vi "HEWH Find Qr and Tmax1.vi"(7 "Water Heater Type":T6, 8 "error in (no error)":errorcluster, 11 "UEF Calculated Values":T1 {"Data Indexes"."15 sec after Draw Index" format="%#.2f"; "Data Indexes"."15 sec after Draw Timestamp" format="%#.2f"; "Data Indexes"."Test Start Timestamp" format="%.2f"; "Data Indexes"."Test End Timestamp" format="%.2f"; "Data Indexes"."T0 Timestamp" format="%.2f"; "Data Indexes"."Tsf Timestamp" format="%.2f"; "Data Indexes"."Tsu0 Timestamp" format="%.2f"; "Data Indexes"."Tmax1 Timestamp" format="%.2f"; "Data Indexes"."Draw Index Timestamp" format="%#.2f"; "Data Indexes"."Non-Draw Timestamp" format="%#.2f"; "Data Indexes"."Heating Timestamp" format="%#.2f"; "Data Indexes"."Start Energy (BTU-Gas)" format="%.6f"; "Data Indexes"."Start Watt Hours" format="%.6f"; "Static Data"."V - Volume of Wh (True)" format="%.5f"; "Static Data"."T-Ambinet Nominal (°F)" format="%.5f"; "Static Data"."T-Inlet Setpoint (°F)" format="%.5f"; "Static Data"."T-Wh Setpoint (°F)" format="%.5f"; "Sampled Data"."Qe (Wh)" format="%.5f"; "Sampled Data"."Tau stby2 (hr)" format="%.5f"; "Sampled Data"."Tastby2 (°F)" format="%.5f"; "Sampled Data"."Qf (BTU)" format="%.5f"; "Sampled Data"."Qe (BTU)" format="%.5f"; "Sampled Data"."Tmax1 (°F)" format="%.5f"; "Sampled Data"."T0 (°F)" format="%.5f"; "Sampled Data"."Qr (BTU)" format="%.5f"; "Sampled Data"."T 24(°F)" format="%.5f"; "Sampled Data"."T astby(°F)" format="%.5f"; "Sampled Data"."T tstby(°F)" format="%.5f"; "Sampled Data"."T su0(°F)" format="%.5f"; "Sampled Data"."T suf(°F)" format="%.5f"; "Sampled Data"."Tau stby_1 (hr)" format="%.5f"; "Sampled Data"."Qsuf (BTU)" format="%.5f"; "Sampled Data"."Qsu0 (BTU)" format="%.5f"; "Calculated Values"."Draw Bonus Volume (gal)" format="%.6f"; "Calculated Values"."Adjustment Factor" format="%.6f"; "Calculated Values"."T*avg_del(n-1)" format="%.6f"; "Calculated Values"."T*min(n-1)" format="%.6f"; "Calculated Values"."T*avg_del(n)" format="%.6f"; "Calculated Values"."Vn" format="%.6f"; "Calculated Values"."Qdm (BTU)" format="%.6f"; "Calculated Values"."QHWD (BTU)" format="%.6f"; "Calculated Values"."QHW (BTU)" format="%.6f"; "Calculated Values"."UEF" format="%.6f"; "Calculated Values"."QHW67 (BTU)" format="%.6f"; "Calculated Values"."Qda (BTU)" format="%.6f"; "Calculated Values"."Qd (BTU)" format="%.6f"; "Calculated Values"."Q (BTU)" format="%.6f"; "Calculated Values"."UA (BTU/(hr*F))" format="%.6f"; "Calculated Values"."Qhr (BTU/hr)" format="%.6f"; "Calculated Values"."Qstby (BTU)" format="%.6f"; "Calculated Values"."nu_r" format="%.6f"; "Calculated Values"."CpUEF (BTU/(lb*F))" format="%.6f"; "Calculated Values"."rho_nu (lb/gal)" format="%.6f"; "Calculated Values"."V1- Vol (Gal)" format="%.6f"; "Calculated Values"."M cluster mass removed (lb)" format="%.6f"; "Calculated Values"."Cp theoretical (BTU/(lbm °F))" format="%.6f"; "Calculated Values"."Tin1 - Mean Inlet 1st Cluster (°F)" format="%.6f"; "Calculated Values"."Tdel1-Mean Outlet 1st Cluster(°F)" format="%.6f"; "Calculated Values"."Cp 24 (BTU/(lb*F))" format="%.6f"; "Calculated Values"."Cp standby (BTU/(lb*F))" format="%.6f"; "Calculated Values"."Cp2 (BTU/(lb*F))" format="%.6f"; "Calculated Values"."Cp1 (BTU/(lb*F))" format="%.6f"; "Calculated Values"."rho 24 (lb/gal)" format="%.6f"; "Calculated Values"."rho standby (lb/gal)" format="%.6f"; "Calculated Values"."rho 2 (lb/gal)" format="%.6f"; "Calculated Values"."Density of cold water All (lbm/gal)" format="%#.3g"; "Calculated Values"."CpHW (BTU/(lbm °F))" format="%#.3g"; "Calculated Values"."Density of hot water All (lbm/gal)" format="%#.3g"; "Calculated Values"."Mass of water All (lbm)" format="%#.3f"}) -> (0 "error out":errorcluster, 3 "UEF Calculated Values Output":T1={"Calculated Values"={"Draw Cluster - Actual (Gal)"=[], "Mass of water All (lbm)"=[], "Density of hot water All (lbm/gal)"=[], "CpHW (BTU/(lbm °F))"=[], "rho 2 (lb/gal)"=0.0, "rho standby (lb/gal)"=0.0, "rho 24 (lb/gal)"=0.0, "Cp1 (BTU/(lb*F))"=0.0, "Cp2 (BTU/(lb*F))"=0.0, "Cp standby (BTU/(lb*F))"=0.0, "Cp 24 (BTU/(lb*F))"=0.0, "nu_r"=0.0, "Qstby (BTU)"=0.0, "Qhr (BTU/hr)"=0.0, "UA (BTU/(hr*F))"=0.0, "Q (BTU)"=0.0, "Qd (BTU)"=0.0, "Qda (BTU)"=0.0, "QHW67 (BTU)"=0.0, "UEF"=0.0, "Tdel1-Mean Outlet 1st Cluster(°F)"=0.0, "Tin1 - Mean Inlet 1st Cluster (°F)"=0.0, "Cp theoretical (BTU/(lbm °F))"=0.0, "M cluster mass removed (lb)"=0.0, "V1- Vol (Gal)"=0.0, "Test Data -Start to End (Full Index)"=[], "rho_nu (lb/gal)"=0.0, "Density of cold water All (lbm/gal)"=[], "CpUEF (BTU/(lb*F))"=0.0, "QHW (BTU)"=0.0, "QHWD (BTU)"=0.0, "Qdm (BTU)"=0.0, "FHD-After 1 Hour (String)"=[], "Vn"=0.0, "T*avg_del(n)"=0.0, "Max Location"=0, "T*min(n-1)"=0.0, "T*avg_del(n-1)"=0.0, "Temp Greater than T*min(n-1)"=FALSE, "Adjustment Factor"=0.0, "Draw Bonus Volume (gal)"=0.0, "Flow Type - End Condition"=enum."ForcedDrawAfterHour"}, "Sampled Data"={"Cold Water Draw Amounts-(Gal)"=[14.98, 1.97, 9.0, 8.97, 4.98, 0.98, 0.96, 0.96, 0.96, 1.96, 1.99, 6.98], "T del_all - Outlet Temps (°F)"=[121.5, 121.3, 124.5, 120.0, 121.2, 120.1, 119.0, 120.3, 116.6, 118.8, 118.3, 118.3], "T in_all - Inlet Temps (°F)"=[58.5, 58.2, 58.4, 58.6, 58.6, 58.1, 58.1, 58.3, 56.3, 58.5, 58.5, 58.5], "Qsu0 (BTU)"=9772.3, "Qsuf (BTU)"=9773.0, "Tau stby_1 (hr)"=6.7, "T suf(°F)"=107.7, "T su0(°F)"=109.3, "T tstby(°F)"=108.5, "T astby(°F)"=68.2, "T 24(°F)"=117.9, "Qr (BTU)"=7628.5, "T0 (°F)"=121.1, "Tmax1 (°F)"=122.4, "Qe (BTU)"=29606.3, "Qf (BTU)"=0.0, "Tastby2 (°F)"=68.3, "RTD Out Full Data\nSet (Each Draw)"=[], "RTD IN Full Data\nSet (Each Draw)"=[], "Tau stby2 (hr)"=23.406, "Hot Water Draw Amounts-(Gal)"=[], "Cold Flow Rate (GPM)"=[], "Hot Flow Rate (GPM)"=[], "Softw Elapsed Time\n Full Data Set (Each Draw)"=[], "Cold Gal Total Full\nData Set (Each Draw)"=[], "Total Hot Draw Amount (Gal) "=0.0, "Total Cold Draw Amount (Gal)"=0.0, "Qe (Wh)"=0.0, "Hot Gal Total Full\nData Set (Each Draw)"=[]}, "Static Data"={"T-Wh Setpoint (°F)"=125.0, "T-Inlet Setpoint (°F)"=58.0, "T-Ambinet Nominal (°F)"=67.5, "V - Volume of Wh (True)"=46.0}, "Data Indexes"={"Test Start-Full Index (Found)"=0, "Header Length"=0, "Draw Index (Found)"=[], "Nr"=0, "Start Watt Hours"=0.0, "Tsu0 Index (Found)"=0, "Tsf Index (Found)"=0, "Start Energy (BTU-Gas)"=0.0, "Draws in Cluster"=0, "T0 Index-Full Index (Found)"=0, "Non-Draw Index (Found)"=[], "Tmax1 Index (Found)"=0, "Test End-Full Index (Found)"=0, "Heating Index (Found)"=[], "Heating Timestamp"=[], "Non-Draw Timestamp"=[], "Draw Index Timestamp"=[], "Tmax1 Timestamp"=0.0, "Tsu0 Timestamp"=0.0, "Tsf Timestamp"=0.0, "T0 Timestamp"=0.0, "Test End Timestamp"=0.0, "Test Start Timestamp"=0.0, "15 sec after Draw Timestamp"=[], "15 sec after Draw Index"=[], "Tmax1 Occurred During a Draw"=FALSE, "FHD Total Time (Sec)"=0.0, "Draw Pattern"=enum."Very Small Usage", "Standby Valid"=FALSE}, "Raw Data"={"Elapsed Time Index (DBL)"=0, "Software Elapsed Time Index (DBL)"=0, "TC Tree Avg Index (DBL)"=0, "Watt Hours -Wh Index (DBL)"=0, "Energy BTU Index (DBL)"=0, "Totalized Flow Index (DBL)"=0, "Flow Rate Index (DBL)"=0, "Program Status Index (Str)"=0, "RTDin Index (DBL)"=0, "RTDout Index (DBL)"=0, "RTDamb Index (DBL)"=0, "Test Data-Start to End DBL"=[], "Data Type"=enum."GEA Inlet Side Meter", "Heat Source Index (DBL)"=0, "Hot Water Rate GPM (DBL)"=0, "Hot Water Total - GAL (DBL)"=0, "FHD-After 1 hour"=[], "Humidity -% RH (DBL)"=0, "Voltage - V (DBL)"=0, "Draw Count (DBL)"=0, "Elapsed Time Index (Str)"=0, "Software Elapsed Time Index (Str)"=0, "Frequency-Hz (Str)"=0, "RTDin Index (Str)"=0, "RTDout Index (Str)"=0, "RTDamb Index (Str)"=0, "UE (Str)"=0, "LE (Str)"=0, "Compressor (Str)"=0, "Flow Rate Index (Str)"=0, "Hot Water Total - GAL (Str)"=0}, "Tolerance Check (T)=Pass"={"Flow Rate"=FALSE, "Totalized Flow"=FALSE, "Ambient Temp (Full Range)"=FALSE, "Ambient Humidity (Full Range)"=FALSE, "Inlet Temp"=FALSE, "Outlet Temp"=FALSE, "Valid Test"=FALSE, "Individual Totalized Flow"=FALSE, "Data Sheet Check"="", "Inlet Temperature"=[], "Tinlet Max"=[], "Tinlet Min"=[], "Flow Rate Max (Tol)"=[], "Flow Rate Min (Tol)"=[], "Amb Temp Max"=0.0, "Amb Temp Min"=0.0, "Toutlet Max - Draw 1"=0.0, "Humidity Upper Tolerance (%)"=0.0, "Total Volume Tolerance (Gal)"=0.0, "Humidity Lower Tolerance (%)"=0.0, "Flow Rate Max\nPer Draw"=[], "Flow Rate Min\nPer Draw"=[], "Ambient Humidity (Runtime)"=FALSE, "Humidity Avg (Runtime)"=0.0, "Ambient Temp (On-Time AVG)"=FALSE, "Ambient Temp (Off-Time AVG)"=FALSE, "Amb Temp OFF Avg"=0.0, "Amb Temp ON Avg"=0.0, "Voltage (Heating)"=FALSE, "Voltage (Min)"=0.0, "Voltage (Max)"=0.0, "Toutlet Max"=[], "Toutlet Min"=[], "Test_Avg_Outlet_Temp"=0.0}, "Test Information"={"TR Number"="", "Lab ID"="", "Notes/Config"="", "Model Number"="", "Serial Number"="", "Lab Technician"="", "Engineer"="", "Type of Fuel"="", "Samp Received Date"="", "Samp Test Date"="", "Report Date"="", "Rate Input (kW or BTU/hr)"="", "Measured Input (kW or BTU/hr)"="", "Filename"="", "Calibration Information"=[], "Calculator Version"="", "Minimum UEF Per CFR"=0.0, "UEF Report Information"=[], "FHR Report Information"=[], "FHR Front Panel Display"=[], "UEF Front Panel Display"=[], "Draw Outlet Temp Viewer"=[]}} {"Data Indexes"."15 sec after Draw Index" format="%#.2f"; "Data Indexes"."15 sec after Draw Timestamp" format="%#.2f"; "Data Indexes"."Test Start Timestamp" format="%.2f"; "Data Indexes"."Test End Timestamp" format="%.2f"; "Data Indexes"."T0 Timestamp" format="%.2f"; "Data Indexes"."Tsf Timestamp" format="%.2f"; "Data Indexes"."Tsu0 Timestamp" format="%.2f"; "Data Indexes"."Tmax1 Timestamp" format="%.2f"; "Data Indexes"."Draw Index Timestamp" format="%#.2f"; "Data Indexes"."Non-Draw Timestamp" format="%#.2f"; "Data Indexes"."Heating Timestamp" format="%#.2f"; "Data Indexes"."Start Energy (BTU-Gas)" format="%.6f"; "Data Indexes"."Start Watt Hours" format="%.6f"; "Static Data"."V - Volume of Wh (True)" format="%.5f"; "Static Data"."T-Ambinet Nominal (°F)" format="%.5f"; "Static Data"."T-Inlet Setpoint (°F)" format="%.5f"; "Static Data"."T-Wh Setpoint (°F)" format="%.5f"; "Sampled Data"."Qe (Wh)" format="%.5f"; "Sampled Data"."Tau stby2 (hr)" format="%.5f"; "Sampled Data"."Tastby2 (°F)" format="%.5f"; "Sampled Data"."Qf (BTU)" format="%.5f"; "Sampled Data"."Qe (BTU)" format="%.5f"; "Sampled Data"."Tmax1 (°F)" format="%.5f"; "Sampled Data"."T0 (°F)" format="%.5f"; "Sampled Data"."Qr (BTU)" format="%.5f"; "Sampled Data"."T 24(°F)" format="%.5f"; "Sampled Data"."T astby(°F)" format="%.5f"; "Sampled Data"."T tstby(°F)" format="%.5f"; "Sampled Data"."T su0(°F)" format="%.5f"; "Sampled Data"."T suf(°F)" format="%.5f"; "Sampled Data"."Tau stby_1 (hr)" format="%.5f"; "Sampled Data"."Qsuf (BTU)" format="%.5f"; "Sampled Data"."Qsu0 (BTU)" format="%.5f"; "Calculated Values"."Draw Bonus Volume (gal)" format="%.6f"; "Calculated Values"."Adjustment Factor" format="%.6f"; "Calculated Values"."T*avg_del(n-1)" format="%.6f"; "Calculated Values"."T*min(n-1)" format="%.6f"; "Calculated Values"."T*avg_del(n)" format="%.6f"; "Calculated Values"."Vn" format="%.6f"; "Calculated Values"."Qdm (BTU)" format="%.6f"; "Calculated Values"."QHWD (BTU)" format="%.6f"; "Calculated Values"."QHW (BTU)" format="%.6f"; "Calculated Values"."UEF" format="%.6f"; "Calculated Values"."QHW67 (BTU)" format="%.6f"; "Calculated Values"."Qda (BTU)" format="%.6f"; "Calculated Values"."Qd (BTU)" format="%.6f"; "Calculated Values"."Q (BTU)" format="%.6f"; "Calculated Values"."UA (BTU/(hr*F))" format="%.6f"; "Calculated Values"."Qhr (BTU/hr)" format="%.6f"; "Calculated Values"."Qstby (BTU)" format="%.6f"; "Calculated Values"."nu_r" format="%.6f"; "Calculated Values"."CpUEF (BTU/(lb*F))" format="%.6f"; "Calculated Values"."rho_nu (lb/gal)" format="%.6f"; "Calculated Values"."V1- Vol (Gal)" format="%.6f"; "Calculated Values"."M cluster mass removed (lb)" format="%.6f"; "Calculated Values"."Cp theoretical (BTU/(lbm °F))" format="%.6f"; "Calculated Values"."Tin1 - Mean Inlet 1st Cluster (°F)" format="%.6f"; "Calculated Values"."Tdel1-Mean Outlet 1st Cluster(°F)" format="%.6f"; "Calculated Values"."Cp 24 (BTU/(lb*F))" format="%.6f"; "Calculated Values"."Cp standby (BTU/(lb*F))" format="%.6f"; "Calculated Values"."Cp2 (BTU/(lb*F))" format="%.6f"; "Calculated Values"."Cp1 (BTU/(lb*F))" format="%.6f"; "Calculated Values"."rho 24 (lb/gal)" format="%.6f"; "Calculated Values"."rho standby (lb/gal)" format="%.6f"; "Calculated Values"."rho 2 (lb/gal)" format="%.6f"; "Calculated Values"."Density of cold water All (lbm/gal)" format="%#.3g"; "Calculated Values"."CpHW (BTU/(lbm °F))" format="%#.3g"; "Calculated Values"."Density of hot water All (lbm/gal)" format="%#.3g"; "Calculated Values"."Mass of water All (lbm)" format="%#.3f"})   [LabVIEW 2023]
uses:
  Type Definitions/UEF Constants.ctl
  Type Definitions/HEWH Draw Stats.ctl
  Type Definitions/HEWH FHR Draw Type.ctl
  Type Definitions/FHR Bins.ctl
  Type Definitions/HEWH Meter Type.ctl
  Type Definitions/HEWH Water Heater Type.ctl
panel:
  # "FHR"
  # "FHR"
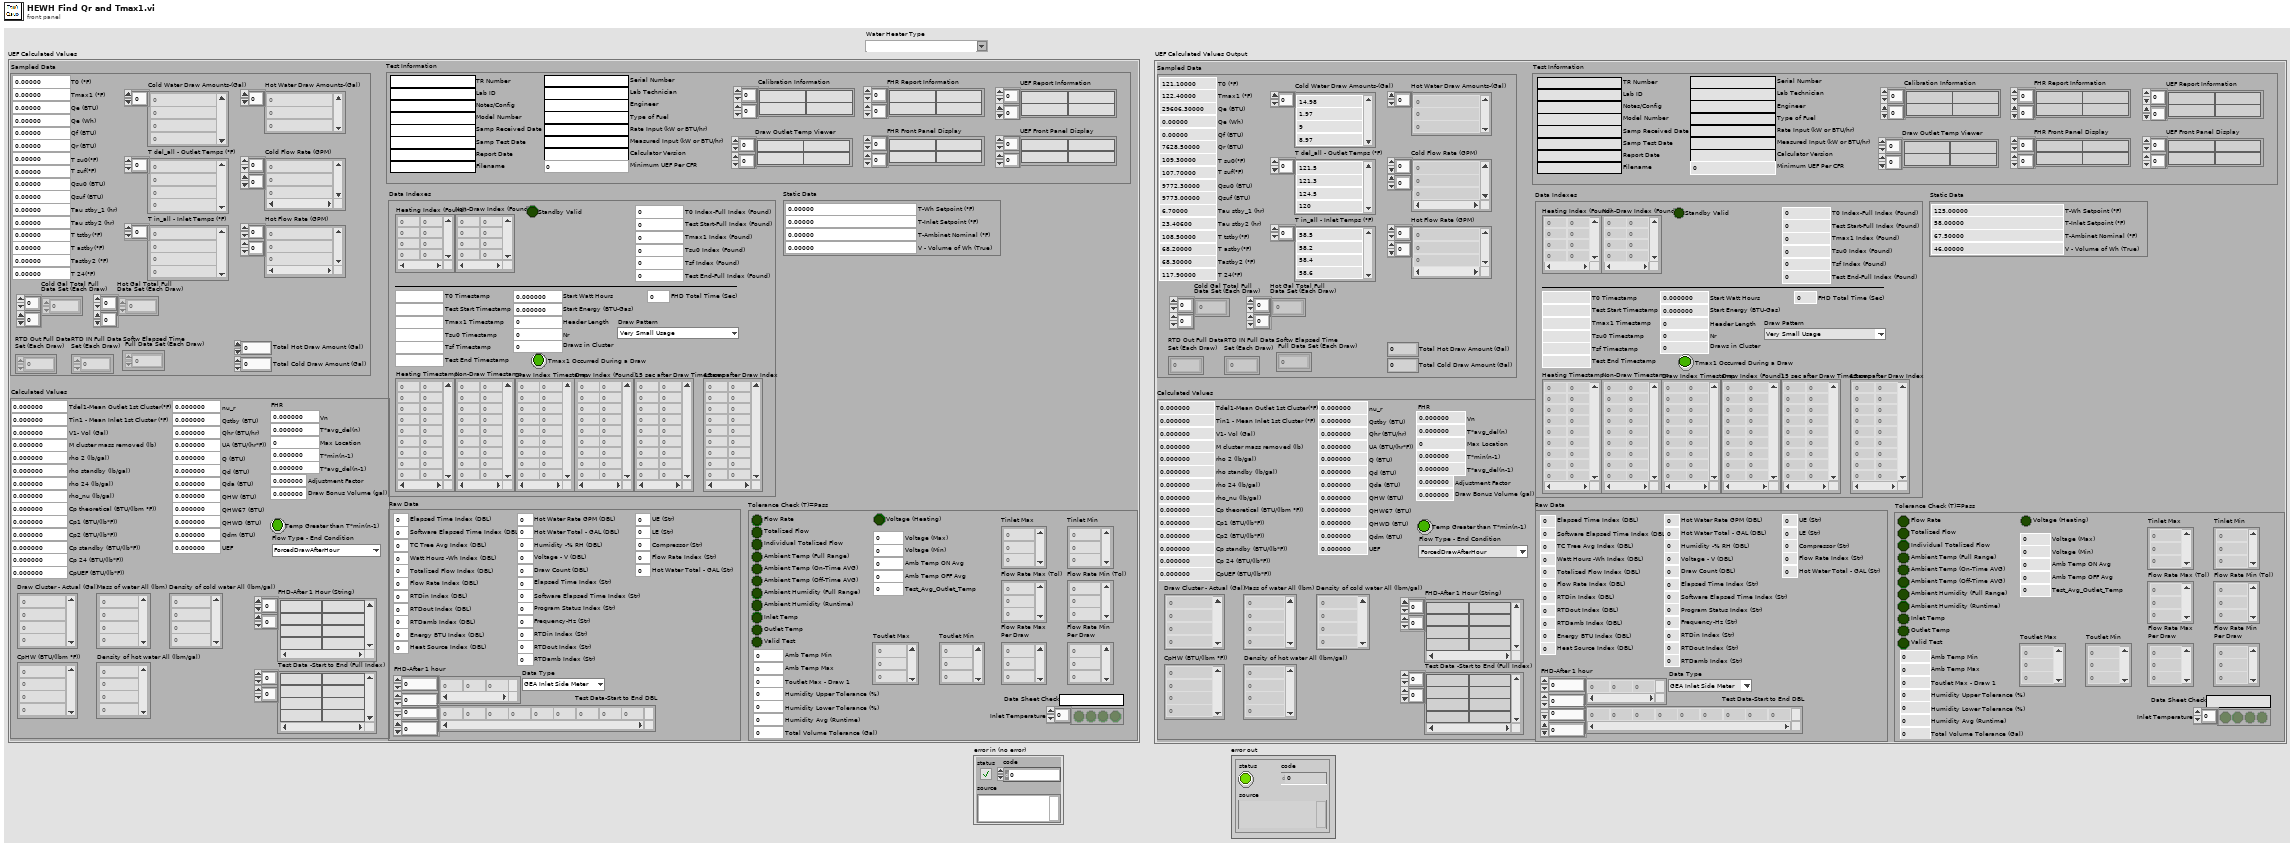
[diagram p1: front panel]
types:
  T1 = typedef "UEF Constants.ctl" = cluster{"Calculated Values":T2, "Sampled Data":cluster{"Cold Water Draw Amounts-(Gal)":dbl[], "T del_all - Outlet Temps (°F)":dbl[], "T in_all - Inlet Temps (°F)":dbl[], "Qsu0 (BTU)":dbl, "Qsuf (BTU)":dbl, "Tau stby_1 (hr)":dbl, "T suf(°F)":dbl, "T su0(°F)":dbl, "T tstby(°F)":dbl, "T astby(°F)":dbl, "T 24(°F)":dbl, "Qr (BTU)":dbl, "T0 (°F)":dbl, "Tmax1 (°F)":dbl, "Qe (BTU)":dbl, "Qf (BTU)":dbl, "Tastby2 (°F)":dbl, "RTD Out Full Data\nSet (Each Draw)":dbl[][], "RTD IN Full Data\nSet (Each Draw)":dbl[][], "Tau stby2 (hr)":dbl, "Hot Water Draw Amounts-(Gal)":dbl[], "Cold Flow Rate (GPM)":dbl[][], "Hot Flow Rate (GPM)":dbl[][], "Softw Elapsed Time\n Full Data Set (Each Draw)":dbl[][], "Cold Gal Total Full\nData Set (Each Draw)":dbl[][], "Total Hot Draw Amount (Gal) ":dbl, "Total Cold Draw Amount (Gal)":dbl, "Qe (Wh)":dbl, "Hot Gal Total Full\nData Set (Each Draw)":dbl[][]}, "Static Data":cluster{"T-Wh Setpoint (°F)":dbl, "T-Inlet Setpoint (°F)":dbl, "T-Ambinet Nominal (°F)":dbl, "V - Volume of Wh (True)":dbl}, "Data Indexes":cluster{"Test Start-Full Index (Found)":i32, "Header Length":i32, "Draw Index (Found)":i32[][], "Nr":i32, "Start Watt Hours":dbl, "Tsu0 Index (Found)":i32, "Tsf Index (Found)":i32, "Start Energy (BTU-Gas)":dbl, "Draws in Cluster":i32, "T0 Index-Full Index (Found)":i32, "Non-Draw Index (Found)":i32[][], "Tmax1 Index (Found)":i32, "Test End-Full Index (Found)":i32, "Heating Index (Found)":i32[][], "Heating Timestamp":dbl[][], "Non-Draw Timestamp":dbl[][], "Draw Index Timestamp":dbl[][], "Tmax1 Timestamp":dbl, "Tsu0 Timestamp":dbl, "Tsf Timestamp":dbl, "T0 Timestamp":dbl, "Test End Timestamp":dbl, "Test Start Timestamp":dbl, "15 sec after Draw Timestamp":dbl[][], "15 sec after Draw Index":dbl[][], "Tmax1 Occurred During a Draw":bool, "FHD Total Time (Sec)":dbl, "Draw Pattern":T4, "Standby Valid":bool}, "Raw Data":cluster{"Elapsed Time Index (DBL)":i32, "Software Elapsed Time Index (DBL)":i32, "TC Tree Avg Index (DBL)":i32, "Watt Hours -Wh Index (DBL)":i32, "Energy BTU Index (DBL)":i32, "Totalized Flow Index (DBL)":i32, "Flow Rate Index (DBL)":i32, "Program Status Index (Str)":i32, "RTDin Index (DBL)":i32, "RTDout Index (DBL)":i32, "RTDamb Index (DBL)":i32, "Test Data-Start to End DBL":dbl[][], "Data Type":T5, "Heat Source Index (DBL)":i32, "Hot Water Rate GPM (DBL)":i32, "Hot Water Total - GAL (DBL)":i32, "FHD-After 1 hour":dbl[][], "Humidity -% RH (DBL)":i32, "Voltage - V (DBL)":i32, "Draw Count (DBL)":i32, "Elapsed Time Index (Str)":i32, "Software Elapsed Time Index (Str)":i32, "Frequency-Hz (Str)":i32, "RTDin Index (Str)":i32, "RTDout Index (Str)":i32, "RTDamb Index (Str)":i32, "UE (Str)":i32, "LE (Str)":i32, "Compressor (Str)":i32, "Flow Rate Index (Str)":i32, "Hot Water Total - GAL (Str)":i32}, "Tolerance Check (T)=Pass":cluster{"Flow Rate":bool, "Totalized Flow":bool, "Ambient Temp (Full Range)":bool, "Ambient Humidity (Full Range)":bool, "Inlet Temp":bool, "Outlet Temp":bool, "Valid Test":bool, "Individual Totalized Flow":bool, "Data Sheet Check":string, "Inlet Temperature":bool[], "Tinlet Max":dbl[], "Tinlet Min":dbl[], "Flow Rate Max (Tol)":dbl[], "Flow Rate Min (Tol)":dbl[], "Amb Temp Max":dbl, "Amb Temp Min":dbl, "Toutlet Max - Draw 1":dbl, "Humidity Upper Tolerance (%)":dbl, "Total Volume Tolerance (Gal)":dbl, "Humidity Lower Tolerance (%)":dbl, "Flow Rate Max\nPer Draw":dbl[], "Flow Rate Min\nPer Draw":dbl[], "Ambient Humidity (Runtime)":bool, "Humidity Avg (Runtime)":dbl, "Ambient Temp (On-Time AVG)":bool, "Ambient Temp (Off-Time AVG)":bool, "Amb Temp OFF Avg":dbl, "Amb Temp ON Avg":dbl, "Voltage (Heating)":bool, "Voltage (Min)":dbl, "Voltage (Max)":dbl, "Toutlet Max":dbl[], "Toutlet Min":dbl[], "Test_Avg_Outlet_Temp":dbl}, "Test Information":cluster{"TR Number":string, "Lab ID":string, "Notes/Config":string, "Model Number":string, "Serial Number":string, "Lab Technician":string, "Engineer":string, "Type of Fuel":string, "Samp Received Date":string, "Samp Test Date":string, "Report Date":string, "Rate Input (kW or BTU/hr)":string, "Measured Input (kW or BTU/hr)":string, "Filename":string, "Calibration Information":string[][], "Calculator Version":string, "Minimum UEF Per CFR":dbl, "UEF Report Information":string[][], "FHR Report Information":string[][], "FHR Front Panel Display":string[][], "UEF Front Panel Display":string[][], "Draw Outlet Temp Viewer":string[][]}}
  T2 = typedef "HEWH Draw Stats.ctl" = cluster{"Draw Cluster - Actual (Gal)":dbl[], "Mass of water All (lbm)":dbl[], "Density of hot water All (lbm/gal)":dbl[], "CpHW (BTU/(lbm °F))":dbl[], "rho 2 (lb/gal)":dbl, "rho standby (lb/gal)":dbl, "rho 24 (lb/gal)":dbl, "Cp1 (BTU/(lb*F))":dbl, "Cp2 (BTU/(lb*F))":dbl, "Cp standby (BTU/(lb*F))":dbl, "Cp 24 (BTU/(lb*F))":dbl, "nu_r":dbl, "Qstby (BTU)":dbl, "Qhr (BTU/hr)":dbl, "UA (BTU/(hr*F))":dbl, "Q (BTU)":dbl, "Qd (BTU)":dbl, "Qda (BTU)":dbl, "QHW67 (BTU)":dbl, "UEF":dbl, "Tdel1-Mean Outlet 1st Cluster(°F)":dbl, "Tin1 - Mean Inlet 1st Cluster (°F)":dbl, "Cp theoretical (BTU/(lbm °F))":dbl, "M cluster mass removed (lb)":dbl, "V1- Vol (Gal)":dbl, "Test Data -Start to End (Full Index)":string[][], "rho_nu (lb/gal)":dbl, "Density of cold water All (lbm/gal)":dbl[], "CpUEF (BTU/(lb*F))":dbl, "QHW (BTU)":dbl, "QHWD (BTU)":dbl, "Qdm (BTU)":dbl, "FHD-After 1 Hour (String)":string[][], "Vn":dbl, "T*avg_del(n)":dbl, "Max Location":i32, "T*min(n-1)":dbl, "T*avg_del(n-1)":dbl, "Temp Greater than T*min(n-1)":bool, "Adjustment Factor":dbl, "Draw Bonus Volume (gal)":dbl, "Flow Type - End Condition":T3}
  T3 = typedef "HEWH FHR Draw Type.ctl" = enum16{"ForcedDrawAfterHour", "HeatingCutoffBeforeHour"}
  T4 = typedef "FHR Bins.ctl" = enum16{"Very Small Usage", "Low Usage", "Medium Usage", "High Usage", "Undefined"}
  T5 = typedef "HEWH Meter Type.ctl" = enum16{"GEA Inlet Side Meter", "GEA Outlet Side Meter", "CSA Inlet Side Meter"}
  T6 = typedef "HEWH Water Heater Type.ctl" = string
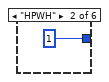
[diagram p2: hidden frame]
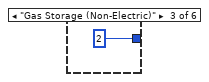
[diagram p3: hidden frame]
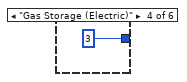
[diagram p4: hidden frame]
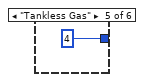
[diagram p5: hidden frame]
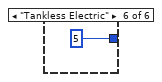
[diagram p6: hidden frame]
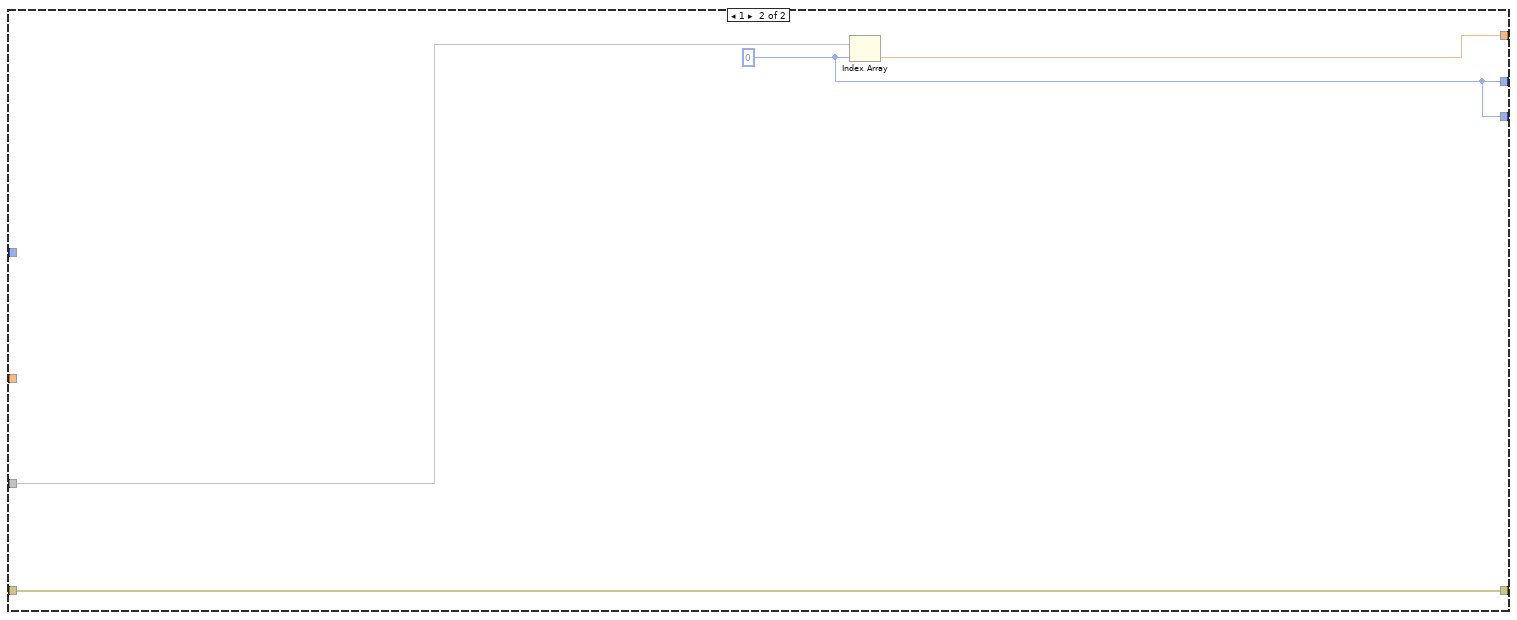
[diagram p8: hidden frame]
diagram:
  # "Find maximum temperature from the \ndraw cluster. This does not include\ndata from the last draw recovery. It stops \nat the last draw"
  # "T¯max,1—maximum measured mean tank temperature after cut-out following the first draw of the 24-hour simulated-use test"
  # "T¯su,0 = the maximum mean tank temperature observed starting five minutes after\nthe first recovery following the final draw of the first draw cluster, °F ( °C)."
  # "Qsu,0 = cumulative energy consumption of the water heater\nfrom the start of the 24-hour simulated-use test to the time\nat which the maximum mean tank temperature is attained starting\nfive minutes after the recovery following the end of the first draw cluster, Btu (kJ)."
  n1 = disable-structure shown="Disabled" {
    disable-tunnel: [w37 _] -> _
    disable-tunnel: [w36 _] -> _
    frame Disabled {
      # "Extract data between a start \nand end point"
      # "Elapsed Time (sec)"
      # "TC Tree Average"
      # "Energy (BTU)"
      # "Watt Hours"
      n2 = formula code="// Inputs:\n// Start_Index: index where to start looking\n// End_Index: index where to stop\n// Elapsed_Time[]: array of timestamps (seconds)\n// Heat_Status[]: array of 0 (OFF) and 1 (ON)\n// Output:\n// Tsuo_Index: index where standby officially starts (after 5 min of heat OFF or post-draw)\n\n// Define Variables\nint32 i;\nfloat Time_RecoveryEnd = -1;\nint32 Tsuo_Index = -1;\nfloat TargetTime;\nfloat Tsuo;\nfloat WH_TO_BTU = 3.41214;   // This is the conversion of Watt-Hours to BTU\nfloat Qsuo_Electric;\nfloat Qsuo_Gas;\n\n//-------- 0.  Skip standby if rated volume < 2 gal  (§5.4.3 applies)\nif (Tank_Volume_Gal < 2) {\n    Tsuo = 0;\n    Tsuo_Index = 0;\n    Tsuo_Software_Elapsed_Time = 0;\n    Qsuo = 0;\n}\n\nelse {\n// Step 1: Look for when heat turns OFF (after being ON)\nfor (i = Start_Index + 1; i <= End_Index; i++) {\n    if (Heat_Status[i - 1] == 1 && Heat_Status[i] == 0) {\n        Time_RecoveryEnd = Elapsed_Time[i];\n        break;\n    }\n}\n\n// Step 2: Determine TargetTime\nif (Time_RecoveryEnd > 0) {\n    // Case 1: Recovery occurred — wait 5 minutes after it ends\n    TargetTime = Time_RecoveryEnd + 300.0;\n} else {\n    // Case 2: No recovery — wait 5 minutes after Start_Index\n    TargetTime = Elapsed_Time[Start_Index] + 300.0;\n}\n\n// Step 3: Find first index where Elapsed_Time >= TargetTime\n// I extract the sofware elapsed time becasue its easier for me to find in the dataset\nfor (i = Start_Index; i <= End_Index; i++) {\n    if (Elapsed_Time[i] >= TargetTime) {\n        Tsuo_Index = i;\n        Tsuo = Test_Data_StartToEnd[Tsuo_Index][TC_Tree_Avg_Index];                                                                     // Extract Tsuo Temp\n        Q_Watt_Hours_Suo = Test_Data_StartToEnd[Tsuo_Index][Watt_Hours_Index];                                             // Extract Watt-Hours \n        Q_EnergyBTU_Index_Suo = Test_Data_StartToEnd[Tsuo_Index][EnergyBTU_Index];                                     // Extract BTU\n        Tsuo_Software_Elapsed_Time = Test_Data_StartToEnd[Tsuo_Index][Software_Elapsed_Time_Index];        // Extract Test Time\n        break;\n    }\n}\n\n// Step 4: Based on the water heater type, evaluate the Qsuo in BTU\nif (Water_Heater_Type == 0) {\n// Calculate Qsuo for Standard Electric and Standard Electronic\nQsuo = Q_Watt_Hours_Suo*WH_TO_BTU;\n}\n\nelse if (Water_Heater_Type == 1) {\n// Calculate Qsuf for HPWH\nQsuo = Q_Watt_Hours_Suo*WH_TO_BTU;\n}\n\nelse if (Water_Heater_Type == 2) {\n// Calculate Qsuf for Gas Storage (Non-Electric)\nQsuo = Q_EnergyBTU_Index_Suo;\n}\n\nelse if (Water_Heater_Type == 3) {\n// Calculate Qsuf for Gas Storage (Electric)\nQsuo_Electric = Q_Watt_Hours_Suo*WH_TO_BTU;\nQsuo_Gas = Q_EnergyBTU_Index_Suo;\n// Add the energy in BTU\nQsuo = Qsuo_Electric + Qsuo_Gas;\n}\n\nelse if (Water_Heater_Type == 4) {\n// Calculate Qsuf for Tankless Gas\nQsuo_Electric = Q_Watt_Hours_Suo*WH_TO_BTU;\nQsuo_Gas = Q_EnergyBTU_Index_Suo;\n// Add the energy in BTU\nQsuo = Qsuo_Electric + Qsuo_Gas;\n}\n\nelse if (Water_Heater_Type == 5) {\n// Calculate Qr for Tankless Electric\nQsuo = Q_Watt_Hours_Suo*WH_TO_BTU;\n}\n\nelse {\n// Default case: Invalid heater type\nQsuo = 0;\n}\n}"() -> ()  [unwired: 11 in, 6 out]
      n3 = formula code="int32 Length;\n\n// If NOT sampling at 5 minutes, increment the start index\nif (takeSampleAt5Min != 1) {\n    StartIndex = StartIndex + 1;\n}\n\n// Calculate how many elements to include in the subset\n// Array Subset uses: (array, start index, length)\nLength = (EndIndex + 1) - StartIndex;"() -> ("StartIndex"=w32:i32, "takeSampleAt5Min"=w31:u8, "Length"=w46:i32)  [unwired: 2 in]
      n4 = Unbundle By Name() -> ("Raw Data.Test Data-Start to End DBL"=w51:dbl[][], "Raw Data.Elapsed Time Index"=w45:i32, "Raw Data.Watt Hours (Wh) Index"=w42:i32, "Raw Data.Energy (BTU) Index"=w43:i32, "Raw Data.TC Tree Avg Index"=w44:i32)  [unwired: 1 in]
      n5 = Index Array(array=w51, index (col)=w45) -> (element=w38:dbl[])  [unwired: 1 in]
      n6 = Index Array(array=w51, index (col)=w42) -> (element=w39:dbl[])  [unwired: 1 in]
      n7 = Index Array(array=w51, index (col)=w43) -> (element=w40:dbl[])  [unwired: 1 in]
      n8 = Index Array(array=w51, index (col)=w44) -> (element=w41:dbl[])  [unwired: 1 in]
      n9 = Array Subset(array=w38, index=w32, length=w46) -> (w47:dbl[])
      n10 = Array Subset(array=w39, index=w32, length=w46) -> (w48:dbl[])
      n11 = Array Subset(array=w40, index=w32, length=w46) -> (w49:dbl[])
      n12 = Array Subset(array=w41, index=w32, length=w46) -> (w50:dbl[])
      n13 = formula code="// Declare variables\nint32 i;                                    // Loop counter\nint32 totalRows;                    // Total number of elements in the ElapsedTimesec array\nfloat T5min;                           // Time threshold, 5 minutes (300 seconds) after first sample\nint32 indexShift5Min;       // Output index of first sample where time exceeds T5min\n\n//  SU0. \nif (takeSampleAt5Min == 1) {\n   indexShift5Min = 0;\n}\nelse {\n// You only do the 5 minute wait for the SUo selection.\n\n// Get the total number of samples (rows) in the ElapsedTimesec array\ntotalRows = sizeOfDim(ElapsedTimesec, 0);\n\n// Set the 5-minute threshold: 300 seconds after the first timestamp\nT5min = ElapsedTimesec[0] + 300;\n\n// Loop through each element in the ElapsedTimesec array\nfor (i = 0; i < totalRows; i++) {\n    // If the current sample time exceeds the 5-minute threshold, exit the loop\n    if (ElapsedTimesec[i] > T5min) {\n        break;   // Stop at the first index that passes the threshold\n    }\n}\n\n// At this point:\n// - If a match was found, 'i' is the first index where ElapsedTimesec[i] > T5min\n// - If no match was found, 'i' will equal totalRows (loop completed without break)\nindexShift5Min = i;\n}"("ElapsedTimesec"=w47, "takeSampleAt5Min"=w31) -> ("indexShift5Min"=w33:i32, "takeSampleAt5Min"=w30:u8)
      n14 = Array Subset(array=w47, index=w33) -> (w34:dbl[])  [unwired: 1 in]
      n15 = Array Subset(array=w48, index=w33) -> (w37:dbl[])  [unwired: 1 in]
      n16 = Array Subset(array=w49, index=w33) -> (w36:dbl[])  [unwired: 1 in]
      n17 = Array Subset(array=w50, index=w33) -> (w35:dbl[])  [unwired: 1 in]
      n18 = case shown="0, Default" w30 {
        tunnel: w35 -> [w75 w98]
        tunnel: w34 -> [w53 _]
        tunnel: [w74 w96] -> _
        tunnel: _ -> [w63 _]
        tunnel: [w62 w95] -> _
        tunnel: w33 -> [w59 _]
        tunnel: [w61 w95] -> _
        tunnel: [w60 w97] -> _
        tunnel: _ -> [w60 w97]
        frame 0, Default {
          # "This is the SUf Index"
          # "Alan calculates this value at 37800-60 seconds. This is exactly correct. The \ndifference comes due to valve open/close in the automated sequence. It takes \napprox. 5-10 seconds. I have been reducing."
          # "Take a look at this. I do not check if the water heater is heating at this point. \n\nIn preparation for determining the energy consumed during standby, record the reading given on the electrical energy (watt-hour) meter, the gas meter,\n and/or the scale used to determine oil consumption, as appropriate. Record the mean tank temperature at the start of the standby period (Tsu,0). At 1-minute\n intervals, record ambient temperature, the electric and/or fuel instrument readings, and the mean tank temperature until the next draw is initiated. The end of\n the standby period is when the final mean tank temperature is recorded, as described. Just prior to initiation of the next draw, record the mean tank temperature\n (Tsu,f). If the water heater is undergoing recovery when the next draw is initiated, record the mean tank temperature (Tsu,f) at the minute prior to the start of the\n recovery. Determine the total electrical energy and/or fossil fuel energy consumption from the beginning of the test to the end of the standby period (Qsu,f). Record\n the time interval between the start of the standby period and the end of the standby period (tstby,1)."
          # "The maximum value of SUo is SUf.\nTherefore, limit this value to SUf\n\nPrevious version used the full array and took the sample\nat 87400 seconds"
          # "I have to wait 5 minutes at the start of the SUo search."
          # "I should probably clean this up and extract the heating source directly. Just like the Elapsed time and TC Tree Avg. \n\nLets get it working first."
          # "Build an array of heating source\nwith the same subset as TC Avg.\nThen strip out the max temp after\n the first heating cycle (if there are \ntwo cycles within the dataset)"
          # "Match time stamps"
          # "Heating source"
          n19 = for {
            tunnel: w53 -> [w76] mode=indexing
            tunnel: [w80] -> w52
            i -> [w80]
            stop <- w81 stop-if-true
            n20 = Subtract(x=37800.0 ("y"), y=60.0) -> (x-y=w77:dbl)
            n21 = Greater Or Equal?(x=w76, y=w77) -> (x >= y?=w81:bool)
          }
          n22 = Unbundle By Name(w63) -> ("Raw Data.Test Data-Start to End DBL"=w64, "Raw Data.Heat Source Index"=w57, "Raw Data.Elapsed Time Index"=w56)
          n23 = Index Array(array=w64, index (col) #1=w57, index (col) #2=w56) -> (element #1=w55, element #2=w54)  [unwired: 2 in]
          n24 = Decrement(x=w52) -> (x-1=w58:i32)
          n25 = Index Array(array=w53, index #1=0 ("index"), index #2=w58) -> (element #1=w66:dbl, element #2=w67:dbl)
          n26 = for {
            tunnel: w54 -> [w94]
            tunnel: w66 -> [w93]
            tunnel: [w91] -> w70
            i -> [w91]
            stop <- w92 stop-if-true
            # "Start Index"
            n27 = Equal?(x=w94, y=w93) -> (x = y?=w92:bool)
          }
          n28 = for {
            tunnel: w54 -> [w90]
            tunnel: w67 -> [w89]
            tunnel: [w87] -> w68
            i -> [w87]
            stop <- w88 stop-if-true
            # "End Index"
            n29 = Equal?(x=w90, y=w89) -> (x = y?=w88:bool)
          }
          n30 = Subtract(x=w68, y=w70) -> (x-y=w69:i32)
          n31 = Increment(x=w69) -> (x+1=w71:i32)
          n32 = Array Subset(array=w55, index=w70, length=w71) -> (w72:void[])
          n33 = for {
            tunnel: w72 -> [w86] mode=indexing
            tunnel: [w83] -> w73 mode=indexing
            tunnel: w75 -> [w83] mode=indexing
            tunnel: [w82] -> _
            i -> [w82]
            stop <- w84 stop-if-true
            # "TC Tree Avg"
            # "Search for the first recovery\nperiod within this dataset"
            n34 = Equal?(x=w86, y=1.0) -> (x = y?=w84:bool)
          }
          n35 = Array Max & Min(array=w73) -> (max value=w74:dbl, max index (indices)=w62:i32)  [unwired: 2 out]
          n36 = Add(x=w62, y=w59) -> (x+y=w61:i32)
        }
        frame 1 {
          w95 = 0 ("index")
          n37 = Index Array(array=w98, index=w95) -> (element=w96:dbl)
        }
      }
      n38 = Add(y=w32) -> ()  [unwired: 1 in, 1 out]
    }
    frame Enabled {
    }
  }
  n39 = Unbundle By Name("UEF Calculated Values") -> ("Raw Data.Test Data-Start to End DBL"=w5:dbl[][], "Raw Data.Elapsed Time Index (DBL)"=w6:i32, "Raw Data.Heat Source Index (DBL)"=w4:i32, "Raw Data.TC Tree Avg Index (DBL)"=w7:i32, "Raw Data.Watt Hours -Wh Index (DBL)"=w19:i32, "Raw Data.Energy BTU Index (DBL)"=w18:i32, "Raw Data.Software Elapsed Time Index (DBL)"=w16:i32, "Static Data.V - Volume of Wh (True)"=w14:dbl, "Data Indexes.Draw Index (Found)"=w13:i32[][], "Data Indexes.Non-Draw Index (Found)"=w12:i32[][], "Data Indexes.Draws in Cluster"=w1:i32, "Data Indexes.Start Watt Hours"=w2:dbl, "Data Indexes.Start Energy (BTU-Gas)"=w3:dbl)
  n40 = case shown="\"Standard Electric\", \"Standard Electronic\", Default" "Water Heater Type" {
    tunnel: [u8 0 u8 1 u8 2 u8 3 u8 4 u8 5] -> w21
    frame "Standard Electric", "Standard Electronic", Default {
    }
    frame "HPWH" {
    }
    frame "Gas Storage (Non-Electric)" {
    }
    frame "Gas Storage (Electric)" {
    }
    frame "Tankless Gas" {
    }
    frame "Tankless Electric" {
    }
  }
  n41 = Index Array(array=w5, index (col)=w6) -> (element=w29:dbl[])  [unwired: 1 in]
  n42 = Index Array(array=w5, index (col)=w4) -> (element=w28:dbl[])  [unwired: 1 in]
  n43 = Index Array(array=w12, index (col) #1=0 ("disabled index (col)"), index (col) #2=1 ("index (col)")) -> (element #1=w11:i32[], element #2=w8:i32[])  [unwired: 2 in]
  n44 = To Unsigned Byte Integer(number=w28) -> (unsigned 8bit integer=w27:u8[])
  n45 = formula code="// --------------------------------------------------------------\n//  LabVIEW Formula-Node  –  Tsuo & Qsu0 capture per 10 CFR 430\n// --------------------------------------------------------------\n//  Inputs (scalars):  Start_Index, End_Index, Tank_Volume_Gal,\n//                     Water_Heater_Type\n//  Inputs (arrays) :  Elapsed_Time[], Heat_Status[],\n//                     TC_Tree_Avg[], Watt_Hours[], Gas_Energy_BTU[],\n//                     Software_Elapsed_Time[], Test_Data_StartToEnd[]\n//\n//  Outputs (scalars): Tsuo_Index, Tsuo, Tsuo_Software_Elapsed_Time, Qsuo\n//----------------------------------------------------------------\n\n//-- Constants\nfloat WH_TO_BTU = 3.41214;\n\n//-- Local variables\nint32  i;\nfloat  DrawEndTime;\nint32  RecoveryWithin5 = 0;\nfloat  Time_RecoveryEnd;\nfloat  TargetTime;\nint32  firstOK;\nint32  candidate;\nfloat  Q_Watt_Hours_Suo;\nfloat  Q_EnergyBTU_Index_Suo;\nint32 Start_Index;\nint32 End_Index;\nint32 Cluster_Last_Draw_Index;\nint32 N;\nint32 j;\n\n//-- Default outputs\nint32 Tsuo_Index                 = -1;\nfloat Tsuo                       = 0.0;\nfloat Tsuo_Software_Elapsed_Time = 0.0;\nfloat Qsuo                       = 0.0;\n\n//---------------------------------------------------------------\n// Get the start and stop indexes, this represents the standby period\n//---------------------------------------------------------------\nCluster_Last_Draw_Index = DrawIndex[LastDrawInCluster - 1][1];\n\nN = sizeOfDim(NonDrawIndexStart, 0);\n\n// Find first NonDrawIndexStart that exceeds the last draw index\nfor (j = 0; j < N; j++) {\n    if (NonDrawIndexStart[j] > Cluster_Last_Draw_Index) {\n        break;                      // j now points at desired window\n    }\n}\n\n// Safety check: did we actually find one?\nif (j < N) {\n    Start_Index = NonDrawIndexStart[j];\n    End_Index   = NonDrawIndexEnd[j];\n} else {\n    // No non-draw window found after the last draw\n    // — handle as needed (error flag, default indices, etc.) —\n    Start_Index = -1;\n    End_Index   = -1;\n}\n\n//---------------------------------------------------------------\n// 0.  Skip standby calculations for units < 2 gal  (§5.4.3)\n//---------------------------------------------------------------\nif (Tank_Volume_Gal < 2.0) {\n    Tsuo       = 0.0;\n    Tsuo_Index = 0;\n    Qsuo       = 0.0;\n}\n\n//---------------------------------------------------------------\n// 0-A. Invalid standby window guard\n//---------------------------------------------------------------\nelse if (Start_Index < 0 || End_Index < 0) {\n    Tsuo       = 0.0;\n    Tsuo_Index = -1;\n    Qsuo       = 0.0;\n}\n\n//---------------------------------------------------------------\n// 1.  Determine correct §5.4.2 branch (recovery vs. no-recovery)\n//---------------------------------------------------------------\nelse {\n\n    DrawEndTime = Elapsed_Time[Start_Index];\n\n    // Look 5 min ahead for any recovery (Heat_Status == 1)\n    for (i = Start_Index; i <= End_Index; i++) {\n        if (Elapsed_Time[i] > DrawEndTime + 300.0) { break; }\n        if (Heat_Status[i] == 1) { RecoveryWithin5 = 1; break; }\n    }\n\n    //-----------------------------------------------------------\n    // 2A. Branch A — recovery occurs within 5 min\n    //-----------------------------------------------------------\n    if (RecoveryWithin5 == 1) {\n\n        // 2A-1. Find OFF edge that ends recovery\n        Time_RecoveryEnd = -1.0;\n        for (i = Start_Index + 1; i <= End_Index; i++) {\n            if (Heat_Status[i - 1] == 1 && Heat_Status[i] == 0) {\n                Time_RecoveryEnd = Elapsed_Time[i];\n                break;\n            }\n        }\n\n        if (Time_RecoveryEnd >= 0.0) {\n            TargetTime = Time_RecoveryEnd + 300.0;        // 5-min gate\n\n            // 2A-2. First sample = TargetTime\n            firstOK = -1;\n            for (i = Start_Index; i <= End_Index; i++) {\n                if (Elapsed_Time[i] >= TargetTime) { firstOK = i; break; }\n            }\n\n            // 2A-3.  Scan forward from firstOK\n            //        • keep the INDEX (candidate) of the highest mean-tank temp\n            //        • stop the scan the moment Heat_Status turns ON\n            if (firstOK >= 0) {\n\n                candidate = firstOK;   // best-so-far index\n\n                for (i = firstOK + 1; i <= End_Index; i++) {\n\n                    /* early exit: recovery has begun */\n                    if (Heat_Status[i] == 1) {\n                        break;                     // leave loop — standby ends here\n                    }\n\n                    /* global-maximum tracker (no separate peakTemp variable) */\n                    if (Test_Data_StartToEnd[i][TC_Tree_Avg_Index] >\n                        Test_Data_StartToEnd[candidate][TC_Tree_Avg_Index]) {\n                        candidate = i;             // new highest temp seen so far\n                    }\n                    /* continue scanning until we hit Heat_Status == 1 or End_Index */\n                }\n                Tsuo_Index = candidate;            // index of true maximum\n            }\n        }\n    }\n\n    //-----------------------------------------------------------\n    // 2B. Branch B — no recovery within 5 min\n    //-----------------------------------------------------------\n    else {\n\n        TargetTime = DrawEndTime + 300.0;               // +5 min exact\n\n        Tsuo_Index = -1;\n        for (i = Start_Index; i <= End_Index; i++) {\n            if (Elapsed_Time[i] >= TargetTime) { Tsuo_Index = i; break; }\n        }\n    }\n\n    //-----------------------------------------------------------\n    // 3.  Stamp Tsuo and cumulative-energy readings (if found)\n    //-----------------------------------------------------------\n    if (Tsuo_Index >= 0) {\n        Tsuo =Test_Data_StartToEnd[Tsuo_Index][TC_Tree_Avg_Index];\n        Tsuo_Software_Elapsed_Time = Test_Data_StartToEnd[Tsuo_Index][Software_Elapsed_Time_Index];\n        Q_Watt_Hours_Suo = (Test_Data_StartToEnd[Tsuo_Index][Watt_Hours_Index])-StartWatt_Hours;\n        Q_EnergyBTU_Index_Suo = (Test_Data_StartToEnd[Tsuo_Index][EnergyBTU_Index])-StartEnergyBTU_Gas;\n\n        //-------------------------------------------------------\n        // 4. Convert Qsuo (Qsu0) to Btu based on heater type\n        //-------------------------------------------------------\n        if (Water_Heater_Type == 0 ||  // Std electric\n            Water_Heater_Type == 1 ||  // HPWH\n            Water_Heater_Type == 5) {  // Tankless electric\n            Qsuo = Q_Watt_Hours_Suo * WH_TO_BTU;\n        }\n        else if (Water_Heater_Type == 2) {               // Gas storage\n            Qsuo = Q_EnergyBTU_Index_Suo;\n        }\n        else if (Water_Heater_Type == 3 ||               // Gas+electric storage\n                 Water_Heater_Type == 4) {               // Tankless gas = 2 gal\n            Qsuo = Q_EnergyBTU_Index_Suo + Q_Watt_Hours_Suo * WH_TO_BTU;\n        }\n        else {                                           // Unknown type\n            Qsuo = 0.0;\n        }\n    }\n}"("Elapsed_Time"=w29, "Heat_Status"=w27, "TC_Tree_Avg_Index"=w7, "Water_Heater_Type"=w21, "Test_Data_StartToEnd"=w5, "Watt_Hours_Index"=w19, "EnergyBTU_Index"=w18, "Software_Elapsed_Time_Index"=w16, "Tank_Volume_Gal"=w14, "NonDrawIndexStart"=w11, "DrawIndex"=w13, "LastDrawInCluster"=w1, "NonDrawIndexEnd"=w8, "StartEnergyBTU_Gas"=w3, "StartWatt_Hours"=w2) -> ("Tsuo_Index"=w23:i32, "Tsuo"=w22:dbl, "Qsuo"=w17:dbl, "Tsuo_Software_Elapsed_Time"=w15:dbl)
  n46 = Bundle By Name(cluster="UEF Calculated Values", "Sampled Data.T su0(°F)"=w22, "Data Indexes.Tsu0 Index (Found)"=w23, "Sampled Data.Qsu0 (BTU)"=w17, "Data Indexes.Tsu0 Timestamp"=w15) -> (→"UEF Calculated Values Output":T1)
  n47 = disable-structure shown="Disabled" {
    frame Disabled {
      n48 = call "HEWH Find Q.vi"() -> ()  [unwired: 10 in, 2 out]
    }
    frame Enabled {
    }
  }
  n49 = disable-structure shown="Disabled" {
    frame Disabled {
      # "Not doing SUf here"
      # "In this case, it is always false"
      n50 = Boolean To (0,1)() -> (0, 1=w106:i16)  [unwired: 1 in]
      n51 = Boolean To (0,1)(Boolean=FALSE ("SUf?")) -> (0, 1=w107:i16)
      n52 = formula code="//This item FirstRecoveryPeriodIndex, is noted as StartIndex in the code\n\nint32 i;\nint32 N;\nint32 EndSearchIndexAdd = 0;\nint32 EndSearchIndex;\nint32 Index;\nfloat TC_Max;\nfloat Time_At_Index;\n\n\n// Determine how many elements are in the TCTreeAverage array\nN = sizeOfDim(TCTreeAverage, 0);\n\n// If SUf mode is active, directly use the indexed value as the max\nif (SUf == 1) {\n    TC_Max = TCTreeAverage[SUfIndex];\n     EndSearchIndex = EndSearchIndexAdd + FirstRecoveryPeriodIndex;\n     Index = SUfIndex + FirstRecoveryPeriodIndex;\n     Time_At_Index = ElapsedTimesec [SUfIndex];\n}\n\n// If SUf is inactive and Qr logic is enabled, find the maximum value\nelse if (SUf == 0 && UseQrLogic == 1) {\n\n    // Handle edge case: array is empty\n    if (N == 0) {\n        TC_Max = 0;  // Default value when no data is present\n    }\n\n    // Initialize maximum to zero\n    TC_Max = 0;\n    EndSearchIndexAdd = 0;\n\n    // Loop through the array to find the maximum value\n    for (i = 0; i < N; i++) {\n        if (TCTreeAverage[i] > TC_Max) {\n            TC_Max = TCTreeAverage[i];  // Update max when higher value found\n            Time_At_Index = ElapsedTimesec [i];   // This is the time at TC Max\n            Index = i + FirstRecoveryPeriodIndex;\n            EndSearchIndex = EndSearchIndexAdd + FirstRecoveryPeriodIndex;\n        }\n    }\n}\n\n// In this case, \nelse if (SUf == 0 && UseQrLogic == 0) {\n\nTC_Max = 0;\n\n\n}"("SUf"=w107, "UseQrLogic"=w106) -> ()  [unwired: 4 in, 4 out]
    }
    frame Enabled {
    }
  }
  n53 = disable-structure shown="Disabled" {
    frame Disabled {
      n54 = Bundle By Name() -> (w108:cluster{})  [unwired: 4 in]
      n55 = call "HEWH T and Q Max.vi"() -> ()  [unwired: 13 in, 7 out]
      n56 = call "HEWH Get Recovery Period.vi"("UEF Calculated Values Output"=w108) -> ("error in (no error)"=w109:errorcluster)  [unwired: 12 in, 2 out]
      n57 = call "HEWH T and Q Extract Data.vi"() -> ()  [unwired: 9 in, 7 out]
      n58 = call "HEWH Build Heating Source Array SUo.vi"() -> ()  [unwired: 7 in, 5 out]
      n59 = call "HEWH Find Qr Indexes.vi"() -> ()  [unwired: 13 in, 3 out]
    }
    frame Enabled {
    }
  }
  "error out" <- "error in (no error)"
